vi "ReadRegister.vi"(7 "Device Address":u8, 8 "error in (no error)":errorcluster, 9 "Register Name":T1=enum."Frame Rate", 10 "Registers Info":map{T1, T2}(c390), 11 "II2COUSB":refnum<class "II2COUSB.lvclass">) -> (0 "error out":errorcluster, 2 "DATA":u8[](array[numeric]), 3 "II2COUSB out":refnum<class "II2COUSB.lvclass">)   [LabVIEW 2020, in "CameraI2COUSB.lvlib" / "CameraDemo.lvclass"]
uses:
  CameraDemo.lvclass
  TypeDef/RegisterName.ctl
  TypeDef/RegisterInfo.ctl
  I2CDriver/II2COUSB/II2COUSB/II2COUSB.lvclass
  I2CDriver/II2COUSB/II2COUSB/I2CFlags.ctl
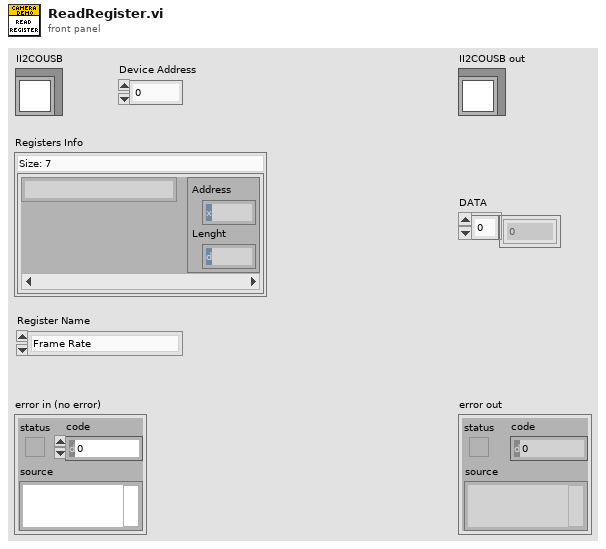
[diagram p1: front panel]
types:
  T1 = typedef "CameraI2COUSB.lvlib/CameraDemo.lvclass/RegisterName.ctl" = enum16{"Clock Rate", "Frame Rate", "Image Type", "Resolution", "Snap", "Start Streaming", "Stop Streaming"}
  T2 = typedef "CameraI2COUSB.lvlib/CameraDemo.lvclass/RegisterInfo.ctl" = cluster{"Address":u16, "Lenght":u32}
  T3 = typedef "II2COUSB.lvlib/II2COUSB.lvclass/I2CFlags.ctl" = u8
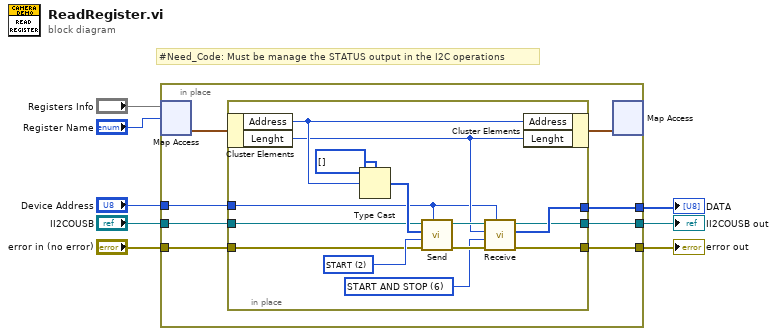
[diagram p0: block diagram]
diagram:
  # "#Need_Code: Must be manage the STATUS output in the I2C operations"
  n1 = in-place {
    in-place-border: "II2COUSB" -> [w15]
    in-place-border: "error in (no error)" -> [w14]
    in-place-border: [w13] -> w3
    in-place-border: "Device Address" -> [w12]
    in-place-border: [w10] -> w2
    in-place-border: [w9] -> w1
    n2 = in-place-map #1("Registers Info", "Register Name") -> (w16:T2)  [unwired: 1 in, 1 out]
    n3 = in-place {
      in-place-border: w15 -> [w20]
      in-place-border: w14 -> [w22]
      in-place-border: [w21] -> w13
      in-place-border: w12 -> [w19]
      in-place-border: [w18] -> w10
      in-place-border: [w17] -> w9
      w24 = T3 6 items=["None"=0, "START"=2, "REPEATED START"=3, "STOP"=4, "START AND STOP"=6] ("eI2Cflags")
      w28 = T3 2 items=["None"=0, "START"=2, "REPEATED START"=3, "STOP"=4, "START AND STOP"=6] ("eI2Cflags")
      n4 = in-place-cluster #2(w16) -> ("Address"=w27:u16, "Lenght"=w23:u32)
      n5 = Type Cast(type=u8[] [], x=w27) -> (*(type *) &x=w29:u8[])
      n6 = call-dynamic "Send.vi"("Device Address"=w19, "error in (no error)"=w22, "eI2Cflags"=w28, "Buffer"=w29, "II2COUSB in"=w20) -> ("error out"=w26:errorcluster, "II2COUSB out"=w25:refnum<class "II2COUSB.lvclass">)  [unwired: 3 in, 2 out]
      n7 = call-dynamic "Receive.vi"("Device Address"=w19, "error in (no error)"=w26, "eI2Cflags"=w24, "Bytes To Read"=w23, "II2COUSB in"=w25) -> ("error out"=w21:errorcluster, "Buffer"=w18:u8[], "II2COUSB out"=w17:refnum<class "II2COUSB.lvclass">)  [unwired: 2 in, 2 out]
      n8 = in-place-cluster #2("Address"=w27, "Lenght"=w23) -> (w11:T2)
    }
    n9 = in-place-map #1(w11) -> ()  [unwired: 1 in, 3 out]
  }
  "error out" <- w3
  "DATA" <- w2
  "II2COUSB out" <- w1
